vi "get_git_hash.vi"(11 "VI folder":string) -> (3 "github hash":string)   [LabVIEW 2014]
uses:
  <vilib>/Utility/file.llb/Read From Spreadsheet File (string).vi
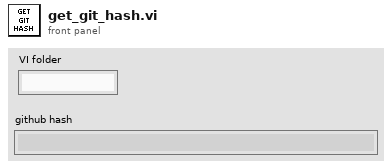
[diagram p1: front panel]
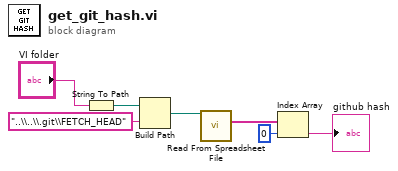
[diagram p0: block diagram]
diagram:
  n1 = String To Path(string="VI folder") -> (path=w1:path)
  n2 = Build Path(base path=w1, name or relative path="..\\..\\.git\\FETCH_HEAD") -> (appended path=w6:path)
  n3 = call-poly <vilib>:"Read From Spreadsheet File.vi"("file path (dialog if empty)"=w6) -> ("first row"=w4:string[])  [unwired: 6 in, 4 out]
  n4 = Index Array(array=w4, index=0) -> (element=→"github hash":string)
